vi "DefineErrorCreationType.vi"(8 "ErrorIn":errorcluster caption="Error In", 10 "ErrorHandlingTypeClass":refnum<class "ErrorCreationExecution.lvclass"> caption="Object In") -> (0 "ErrorOut":errorcluster caption="Error Out")   [LabVIEW 2018, in "ErrorCreationExecution.lvclass"]
uses:
  <userlib>/_express/CustomErrorCreator/ErrorCreationExecution/ErrorCreationExecution.lvclass
  <userlib>/_express/CustomErrorCreator/ErrorCreationExecution/ErrorCreationType.vi
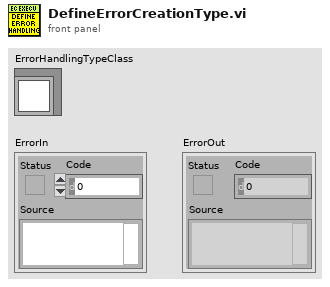
[diagram p1: front panel]
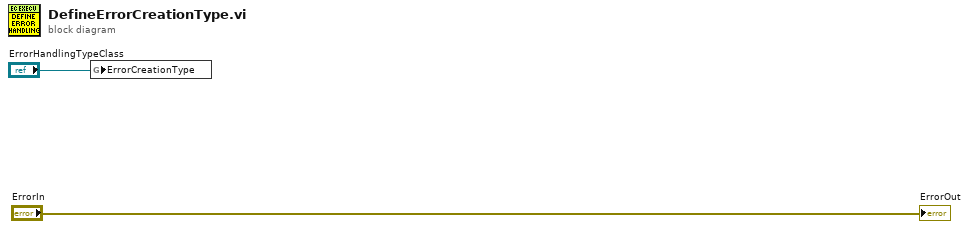
[diagram p0: block diagram]
diagram:
  n1 = global write "ErrorCreationType.vi" "ErrorCreationType"("ErrorHandlingTypeClass") -> ()
  "ErrorOut" <- "ErrorIn"
